vi "Save ROB info to Save File.vi"(8 "error in (no error)":errorcluster, 9 "Fileref":T2 format="%.0x", 11 "ROB info clusters":T1) -> (0 "error out":errorcluster)   [LabVIEW 2016]
uses:
  <vilib>/addons/h5labview2/base/hid_t.ctl
  Typedefs/All ROBs info cluster refnum.ctl
  <vilib>/addons/h5labview2/group/H5G.lvlib
  <vilib>/addons/h5labview2/dataset/H5D.lvlib
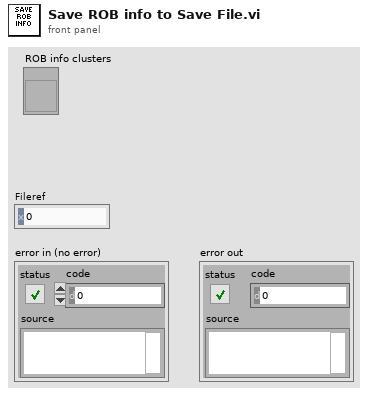
[diagram p1: front panel]
types:
  T1 = typedef "All ROBs info cluster refnum.ctl" = refnum<vi>
  T2 = typedef "hid_t.ctl" = i32
  T3 = enum16{"insertPPS", "insertUTC", "read", "initiate"}
  T4 = cluster{"+5V Rail":sgl, "-5V Rail":sgl, "+3.3V Rail":sgl, "+15V Rail":sgl}
  T5 = enum16{"ID", "Status", "Voltages", "Temp", "Latch count", "VRef", "Trigthres", "MPPC EN?", "Test charge?", "Responding?"}
  T6 = typedef "ROB info refnum.ctl" = refnum<vi>
  T7 = typedef "ROB display info.ctl" = cluster{"ID:":i32, "State:":string, "Voltages":i32, "Temp:":dbl, "Latch count:":i32, "VRef:":enum16{"External", "Internal", "Unknown"}, "Trigthres:":i32, "MPPC EN":bool, "Test charge":bool, "Responding":bool, "Last update":timestamp}
  T8 = cluster{"+5V Rail":sgl, "-5V Rail":sgl, "+3.3V Rail":sgl, "+15V Rail":sgl}[]
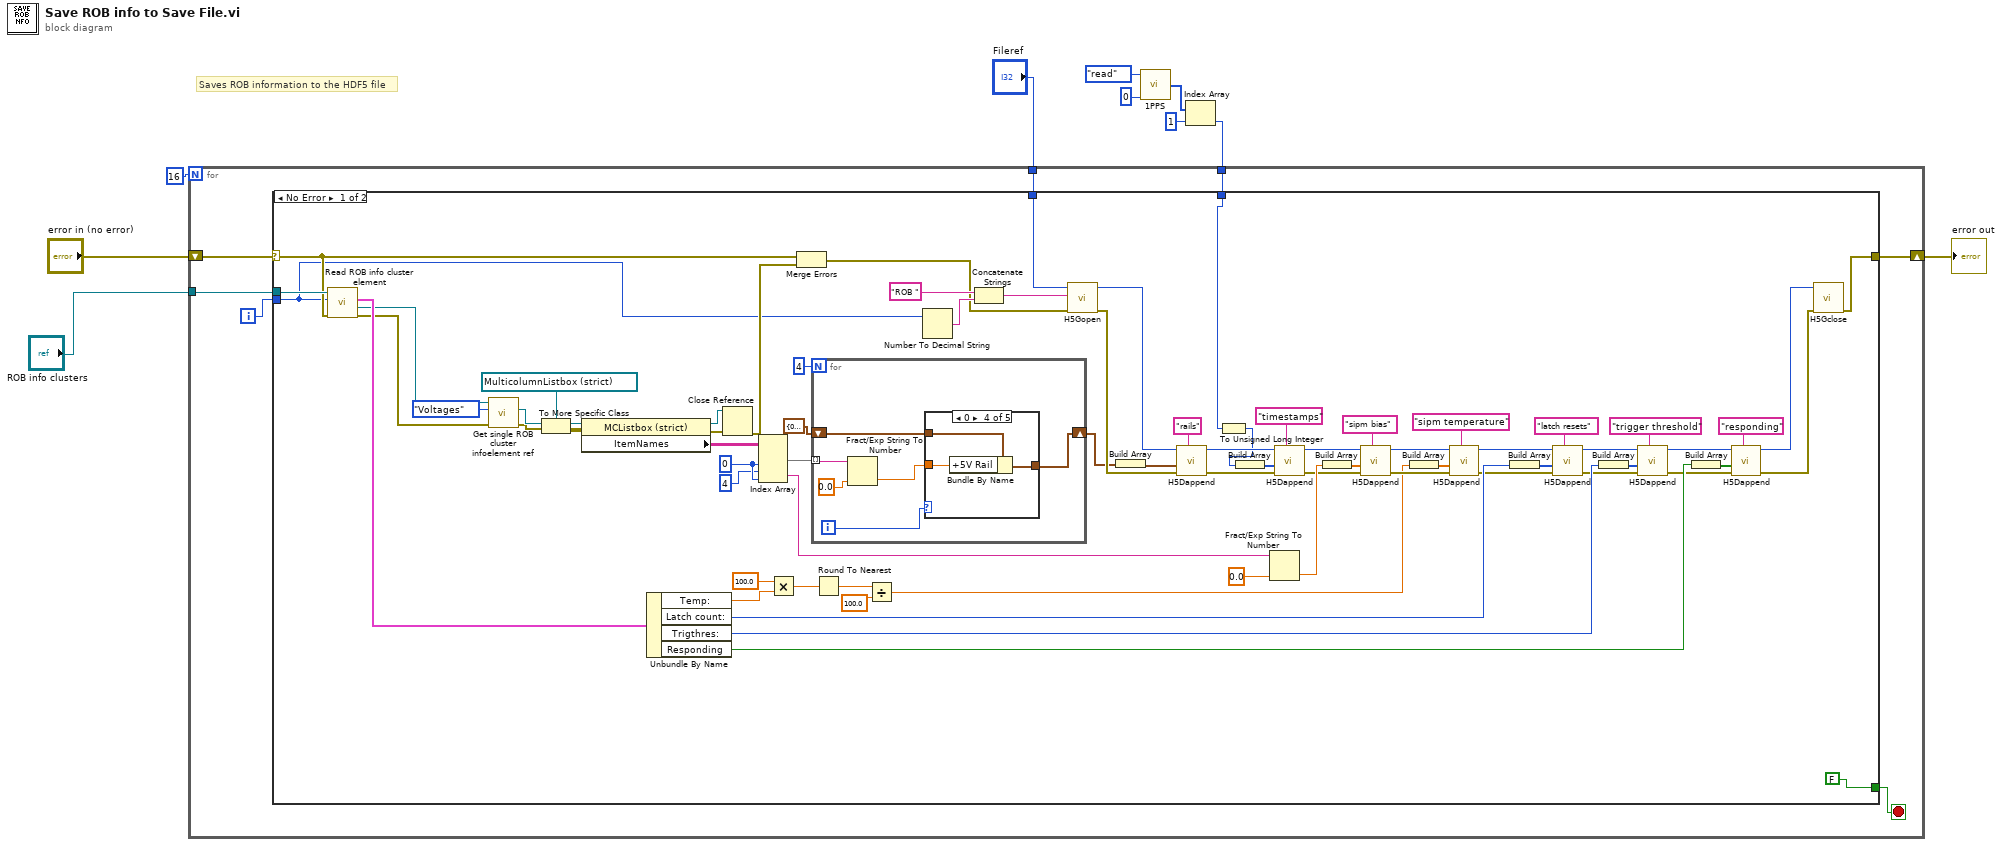
[diagram p0: block diagram]
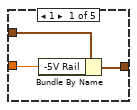
[diagram p2: hidden frame]
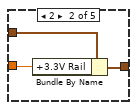
[diagram p3: hidden frame]
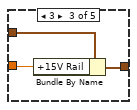
[diagram p4: hidden frame]
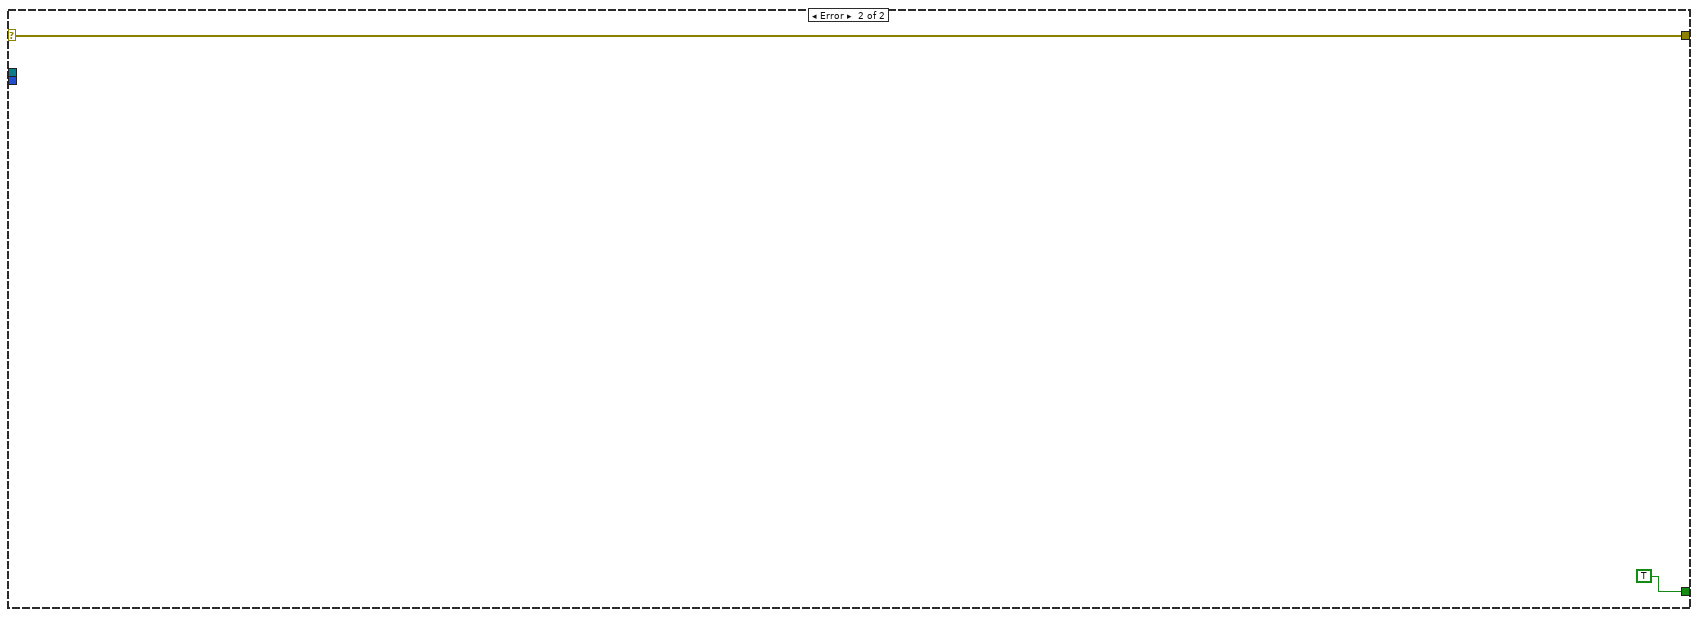
[diagram p6: hidden frame]
diagram:
  # "Saves ROB information to the HDF5 file"
  n1 = call "1PPS.vi"("Read Index\nNumber"=0 ("Read Index\nNumber"), "Action"=T3."read") -> ("Array"=w5:u32[])  [unwired: 2 in]
  n2 = Index Array(array=w5, index=1) -> (element=w4:u32)
  n3 = for {
    N: 16 -> [_]
    tunnel: "ROB info clusters" -> [w17]
    tunnel: w4 -> [w15]
    tunnel: "Fileref" -> [w14]
    shift-right: [w13] -> w10
    shift-left: "error in (no error)" -> [w12]
    i -> [w16]
    stop <- w11 stop-if-true
    n4 = case shown="No Error" w12 {
      selector: w12 -> [w69 w111]
      tunnel: w17 -> [w90 _]
      tunnel: w16 -> [w68 _]
      tunnel: w15 -> [w18 _]
      tunnel: w14 -> [w66 _]
      tunnel: [w65 w111] -> w13
      tunnel: [FALSE TRUE] -> w11
      frame No Error {
        w28 = 0 ("disabled index (col)")
        n5 = call "Read ROB info cluster element.vi"("error in (no error)"=w69, "Channel"=w68, "ROB info clusters"=w90) -> ("error out"=w87:errorcluster, "ROB infocluster ref"=w88:T6, "ROB Info-display"=w89:T7)  [unwired: 5 in, 1 out]
        n6 = call "Get single ROB cluster infoelement ref.vi"("error in (no error)"=w87, "Enum"=T5."Voltages", "ROB infocluster ref"=w88) -> ("error out"=w82:errorcluster, "Element reference"=w85:refnum<vi>)  [unwired: 6 in, 1 out]
        n7 = To More Specific Class(target class=refnum<vi> refnum ("Voltages"), reference=w85, error in=w82) -> (specific class reference=w84:refnum<vi>, error out=w81:errorcluster)
        n8 = property class="MCListbox (strict)"(reference=w84, error in=w81) -> (reference out=w73:refnum<vi>, error out=w74:errorcluster, "ItemNames"=w80:string[][])
        n9 = Unbundle By Name(w89) -> ("Temp:"=w26:dbl, "Latch count:"=w46:i32, "Trigthres:"=w44:i32, "Responding"=w42:bool)
        n10 = Close Reference(reference=w73, error in (no error)=w74) -> (error out=w72:errorcluster)
        n11 = Index Array(array=w80, index (col) #1=w28, index (row) #2=4 ("disabled index (col)"), index (col) #2=w28) -> (element #1=w79:string[], element #2=w75:string)  [unwired: 1 in]
        n12 = Multiply(x=100.0, y=w26) -> (x*y=w24:dbl)
        n13 = Merge Errors(w69, w72) -> (w71:errorcluster)
        n14 = for {
          N: 4 -> [_]
          tunnel: w79 -> [w96] mode=indexing
          shift-right: [w93] -> w56
          shift-left: T4 {"+5V Rail"=0.0, "-5V Rail"=0.0, "+3.3V Rail"=0.0, "+15V Rail"=0.0} -> [w94]
          i -> [w91]
          n15 = Fract/Exp String To Number(string=w96, default (0 dbl)=sgl 0.0 ("+5V Rail")) -> (number=w92:sgl)  [unwired: 2 in, 1 out]
          n16 = case shown="0" w91 {
            tunnel: w94 -> [w98 w101 w104 w108 w109]
            tunnel: [w99 w102 w105 w107 w109] -> w93
            tunnel: w92 -> [w97 w100 w103 w106 _]
            frame 1 {
              n17 = Bundle By Name(cluster=w98, "-5V Rail"=w97) -> (w99:T4)
            }
            frame 2 {
              n18 = Bundle By Name(cluster=w101, "+3.3V Rail"=w100) -> (w102:T4)
            }
            frame 3 {
              n19 = Bundle By Name(cluster=w104, "+15V Rail"=w103) -> (w105:T4)
            }
            frame 0 {
              n20 = Bundle By Name(cluster=w108, "+5V Rail"=w106) -> (w107:T4)
            }
            frame Default {
            }
          }
        }
        n21 = Round To Nearest(number=w24) -> (nearest integer value=w23:dbl)
        n22 = Divide(x=w23, y=100.0) -> (x/y=w21:dbl)
        n23 = Number To Decimal String(number=w68) -> (decimal integer string=w77:string)  [unwired: 1 in]
        n24 = Concatenate Strings("ROB " ("name"), w77) -> (w67:string)
        n25 = call <vilib>:"H5Gopen.vi"("error in (no error)"=w71, "name"=w67, "ref in"=w66) -> ("error out"=w63:errorcluster, "group out"=w58:T2)  [unwired: 7 in]
        n26 = Build Array(w56) -> (w62:T8)
        n27 = call <vilib>:"H5Dappend.vi"("dataset name"="rails" ("name"), "error in (no error)"=w63, "data"=w62, "ref in"=w58) -> ("error out"=w60:errorcluster, "ref out"=w57:T2)  [unwired: 4 in, 2 out]
        n28 = To Unsigned Long Integer(number=w18) -> (unsigned 32bit integer=w19:u32)
        n29 = Build Array(w19) -> (w59:u32[])
        n30 = Fract/Exp String To Number(string=w75, default (0 dbl)=sgl 0.0 ("+5V Rail")) -> (number=w49:sgl)  [unwired: 2 in, 1 out]
        n31 = call <vilib>:"H5Dappend.vi"("dataset name"="timestamps" ("name"), "error in (no error)"=w60, "data"=w59, "ref in"=w57) -> ("error out"=w40:errorcluster, "ref out"=w34:T2)  [unwired: 4 in, 2 out]
        n32 = Build Array(w49) -> (w48:sgl[])
        n33 = call <vilib>:"H5Dappend.vi"("dataset name"="sipm bias" ("name"), "error in (no error)"=w40, "data"=w48, "ref in"=w34) -> ("error out"=w39:errorcluster, "ref out"=w33:T2)  [unwired: 4 in, 2 out]
        n34 = Build Array(w21) -> (w47:dbl[])
        n35 = call <vilib>:"H5Dappend.vi"("dataset name"="sipm temperature" ("name"), "error in (no error)"=w39, "data"=w47, "ref in"=w33) -> ("error out"=w38:errorcluster, "ref out"=w32:T2)  [unwired: 4 in, 2 out]
        n36 = Build Array(w46) -> (w45:i32[])
        n37 = call <vilib>:"H5Dappend.vi"("dataset name"="latch resets" ("name"), "error in (no error)"=w38, "data"=w45, "ref in"=w32) -> ("error out"=w37:errorcluster, "ref out"=w31:T2)  [unwired: 4 in, 2 out]
        n38 = Build Array(w44) -> (w43:i32[])
        n39 = call <vilib>:"H5Dappend.vi"("dataset name"="trigger threshold" ("name"), "error in (no error)"=w37, "data"=w43, "ref in"=w31) -> ("error out"=w36:errorcluster, "ref out"=w30:T2)  [unwired: 4 in, 2 out]
        n40 = Build Array(w42) -> (w41:bool[])
        n41 = call <vilib>:"H5Dappend.vi"("dataset name"="responding" ("name"), "error in (no error)"=w36, "data"=w41, "ref in"=w30) -> ("error out"=w35:errorcluster, "ref out"=w29:T2)  [unwired: 4 in, 2 out]
        n42 = call <vilib>:"H5Gclose.vi"("error in (no error)"=w35, "group in"=w29) -> ("error out"=w65:errorcluster)  [unwired: 9 in]
      }
      frame Error {
      }
    }
  }
  "error out" <- w10
